vi "SMTP Email Escape Periods and ExtChars.vi"(1 "string":string) -> (0 "quoted string":string)   [LabVIEW 2011, in "NewNI_SMTPEmail.lvlib"]
uses:
  NewNI_SMTPEmail.lvlib
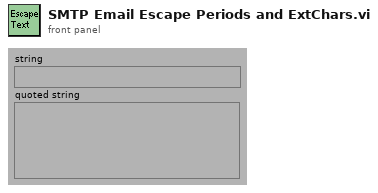
[diagram p1: front panel]
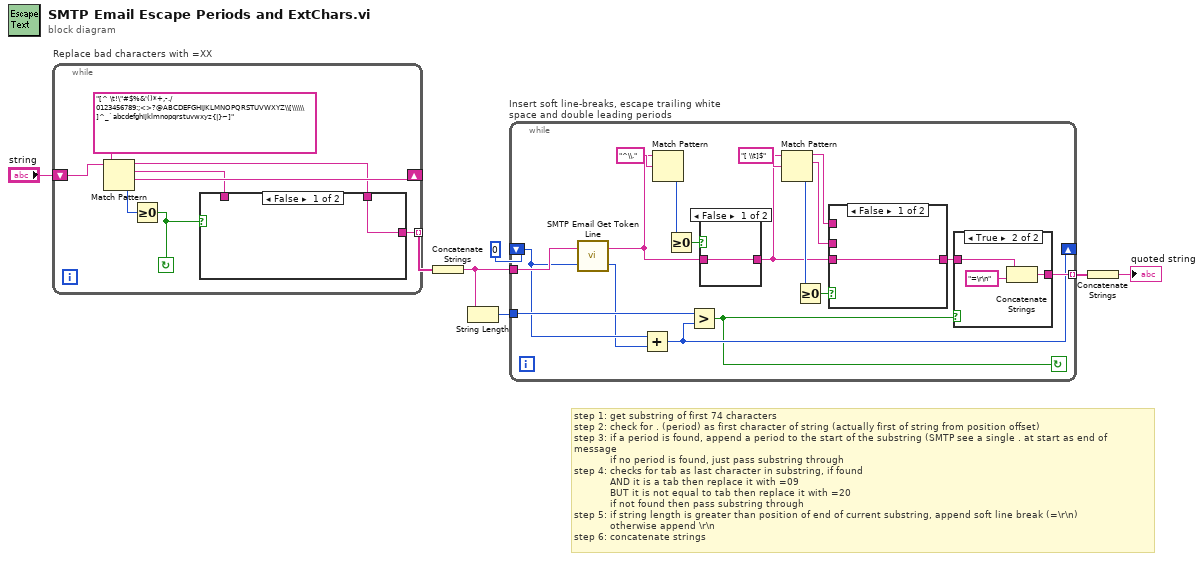
[diagram p0: block diagram]
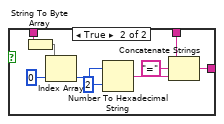
[diagram p2: hidden frame]
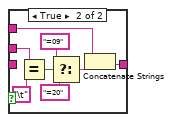
[diagram p3: hidden frame]
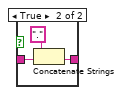
[diagram p4: hidden frame]
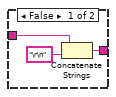
[diagram p5: hidden frame]
diagram:
  # "step 1: get substring of first 74 characters\nstep 2: check for . (period) as first character of string (actually first of string from position offset)\nstep 3: if a period is found, append a period to the start of the substring (SMTP see a single . at start as end of message\n            if no period is found, just pass substring through\nstep 4: checks for tab as last character in substring, if found\n            AND it is a tab then replace it with =09\n            BUT it is not equal to tab then replace it with =20\n            if not found then pass substring through\nstep 5: if string length is greater than position of end of current substring, append soft line break (=\\r\\n)\n            otherwise append \\r\\n\nstep 6: concatenate strings"
  n1 = while "Replace bad characters with =XX" {
    tunnel: [w8] -> w6 mode=indexing
    shift-left: "string" -> [w13]
    shift-right: [w12] -> _
    stop <- w11 continue-if-true
    n2 = Match Pattern(string=w13, regular expression="[^ \t!\"#$%&'()*+,-./0123456789:;<>?@ABCDEFGHIJKLMNOPQRSTUVWXYZ\\[\\\\\\]^_`abcdefghijklmnopqrstuvwxyz{|}~]") -> (before substring=w9:string, match substring=w10:string, after substring=w12:string, offset past match=w14:i32)  [unwired: 1 out]
    n3 = Greater Or Equal To 0?(x=w14) -> (x >= 0?=w11:bool)
    n4 = case shown="False" w11 {
      tunnel: w10 -> [_ w25]
      tunnel: w9 -> [w16 w20]
      tunnel: [w16 w17] -> w8
      frame False {
      }
      frame True {
        n5 = String To Byte Array(string=w25) -> (unsigned byte array=w24:u8[])
        n6 = Index Array(array=w24, index=0) -> (element=w22:u8)
        n7 = Number To Hexadecimal String(1:i16 2 ("width (-)"), 2:w22) -> (0:w19:string)
        n8 = Concatenate Strings(w20, "=", w19) -> (w17:string)
      }
    }
  }
  n9 = Concatenate Strings(w6) -> (w2:string)
  n10 = String Length(string=w2) -> (length=w3:i32)
  n11 = while "Insert soft line-breaks, escape trailing white space and double leading periods" {
    tunnel: w3 -> [w42]
    tunnel: [w43] -> w5 mode=indexing
    shift-left: 0 -> [w28]
    shift-right: [w41] -> _
    tunnel: w2 -> [w29]
    stop <- w40 continue-if-true
    n12 = call "SMTP Email Get Token Line.vi"("Offset"=w28, "string"=w29) -> ("line len"=w26:i32, "Line"=w27:string)
    n13 = Add(x=w28, y=w26) -> (x+y=w41:i32)
    n14 = Match Pattern(string=w27, regular expression="^\\.") -> (offset past match=w38:i32)  [unwired: 4 out]
    n15 = Greater Or Equal To 0?(x=w38) -> (x >= 0?=w37:bool)
    n16 = Greater?(x=w42, y=w41) -> (0:w40:bool)
    n17 = case shown="False" w37 {
      tunnel: w27 -> [w53 w56]
      tunnel: [w53 w55] -> w33
      frame False {
      }
      frame True {
        n18 = Concatenate Strings(".", w56) -> (w55:string)
      }
    }
    n19 = Match Pattern(string=w33, regular expression="[ \\t]$") -> (before substring=w31:string, match substring=w30:string, offset past match=w35:i32)  [unwired: 2 out]
    n20 = Greater Or Equal To 0?(x=w35) -> (x >= 0?=w34:bool)
    n21 = case shown="False" w34 {
      tunnel: w33 -> [w44 _]
      tunnel: [w44 w52] -> w32
      tunnel: w31 -> [_ w51]
      tunnel: w30 -> [_ w50]
      frame False {
      }
      frame True {
        n22 = Equal?(x=w50, y="\t") -> (x = y?=w48:bool)
        n23 = Select(t="=09", s=w48, f="=20") -> (s? t:f=w46:string)
        n24 = Concatenate Strings(w51, w46) -> (w52:string)
      }
    }
    n25 = case shown="True" w40 {
      tunnel: w32 -> [w59 w62]
      tunnel: [w57 w60] -> w43
      frame False {
        n26 = Concatenate Strings(w59, "\r\n") -> (w57:string)
      }
      frame True {
        n27 = Concatenate Strings(w62, "=\r\n") -> (w60:string)
      }
    }
  }
  n28 = Concatenate Strings(w5) -> (→"quoted string":string)
